vi "Find Focus Max.vi"(2 "Averaged Ratio":cluster{"Frequency Array":dbl[], dbl[]}(graph)) -> (6 "Value of Z for max counts":dbl)   [LabVIEW 2014]
panel:
  out "Index of max counts":i32
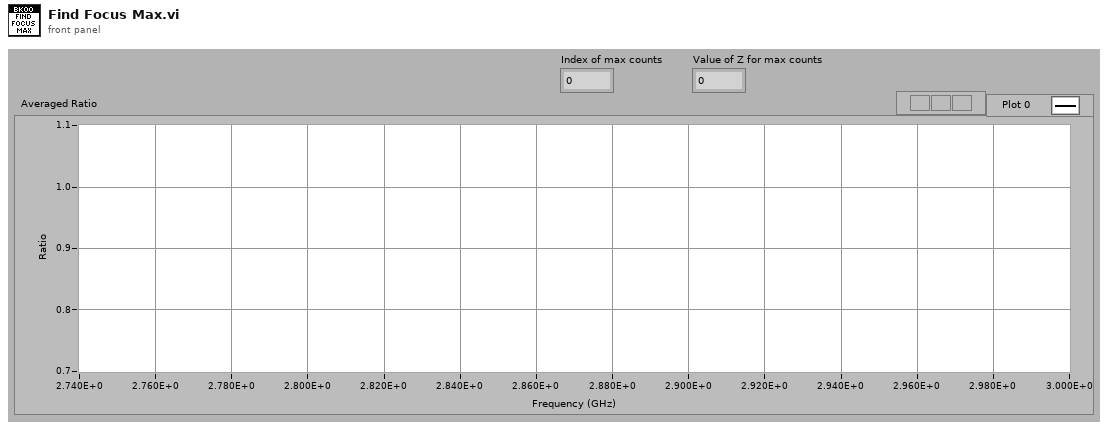
[diagram p1: front panel]
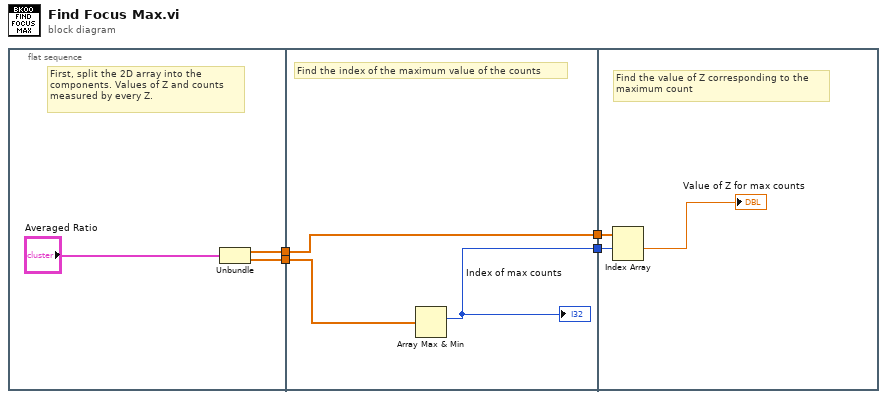
[diagram p0: block diagram]
diagram:
  n1 = flat-sequence {
    tunnel: [w6] -> w4
    tunnel: [w5] -> w1
    tunnel: w4 -> [w10]
    tunnel: [w9] -> w3
    tunnel: [w8] -> w2
    tunnel: w1 -> [w8]
    tunnel: w3 -> [w13]
    tunnel: w2 -> [w11]
    frame #0 {
      # "First, split the 2D array into the \ncomponents. Values of Z and counts\nmeasured by every Z."
      n2 = Unbundle("Averaged Ratio") -> ("Frequency Array"=w5:dbl[], w6:dbl[])
    }
    frame #1 {
      # "Find the index of the maximum value of the counts"
      n3 = Array Max & Min(array=w10) -> (max index (indices)=w9:i32)  [unwired: 3 out]
      "Index of max counts" <- w9
    }
    frame #2 {
      # "Find the value of Z corresponding to the\nmaximum count"
      n4 = Index Array(array=w11, index #1=w13) -> (element #1=→"Value of Z for max counts":dbl)  [unwired: 1 in, 1 out]
    }
  }
